vi "tb_magnitude_power_scalable_host.vi"() -> ()   [LabVIEW 2011]
panel:
  out "FLP":dbl
  out "FXP":dbl
  out "Pass":bool
  in  "Error Margin":dbl=1e-06 format="%#_p"
  out "Error":dbl format="%#_6p"
  in  "Imag":fxp<+/-,18,1>=0.1999969482421875 format="%.18g"
  in  "Real":fxp<+/-,18,1>=0.09999847412109375 format="%.18g"
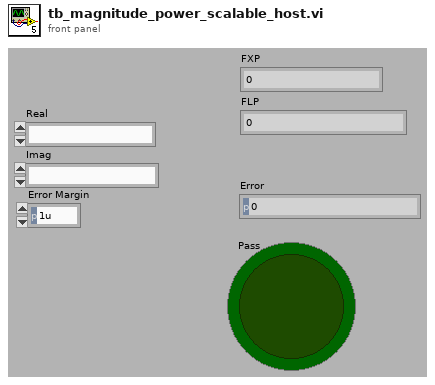
[diagram p1: front panel]
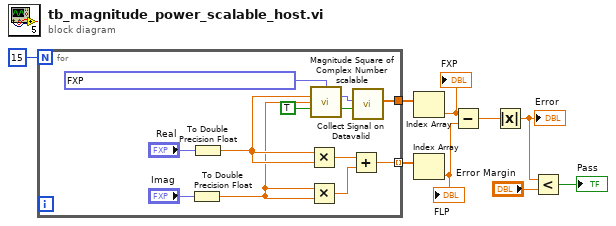
[diagram p0: block diagram]
diagram:
  n1 = for {
    N: 15 -> [_]
    tunnel: [w13] -> w8
    tunnel: [w12] -> w7 mode=indexing
    n2 = To Double Precision Float(number="Imag") -> (double precision float=w10:dbl)
    n3 = To Double Precision Float(number="Real") -> (double precision float=w11:dbl)
    n4 = Multiply(x=w11, y=w11) -> (x*y=w15:dbl)
    n5 = Multiply(x=w10, y=w10) -> (x*y=w14:dbl)
    n6 = call "Magnitude Square of Complex Number scalable.vi"("output type"=fxp<+,37,2> 0.0, "Real"=w11, "Imaginary"=w10, "Input Valid"=TRUE) -> ("Magnitude^2"=w19:fxp<+,37,2>, "Output Valid"=w18:bool)  [unwired: 10 in]
    n7 = Add(x=w15, y=w14) -> (x+y=w12:dbl)
    n8 = call <userlib>:"Collect Signal on Datavalid.vi"("Data Valid"=w18, "Input"=w19) -> ("Output"=w13:dbl[])  [unwired: 9 in]
  }
  n9 = Index Array(array=w8) -> (element=w6:dbl)  [unwired: 1 in]
  "FXP" <- w6
  n10 = Index Array(array=w7) -> (element=w5:dbl)  [unwired: 1 in]
  "FLP" <- w5
  n11 = Subtract(x=w6, y=w5) -> (x-y=w4:dbl)
  n12 = Absolute Value(x=w4) -> (abs(x)=w1:dbl)
  "Error" <- w1
  n13 = Less?(x=w1, y="Error Margin") -> (x < y?=→"Pass":bool)
